vi "Get V.vi"(8 "error in (no error)":errorcluster, 10 "chan (0)":i32, 11 "VISA resource name":refnum<visa-resource-name>) -> (0 "error out":errorcluster, 2 "output":string, 3 "VISA resource name out":refnum<visa-resource-name>)   [LabVIEW 2023]
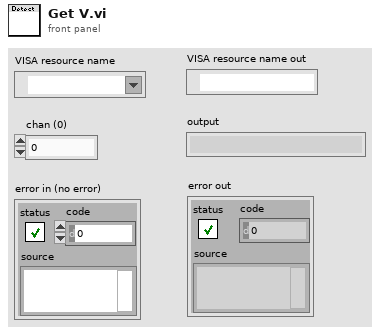
[diagram p1: front panel]
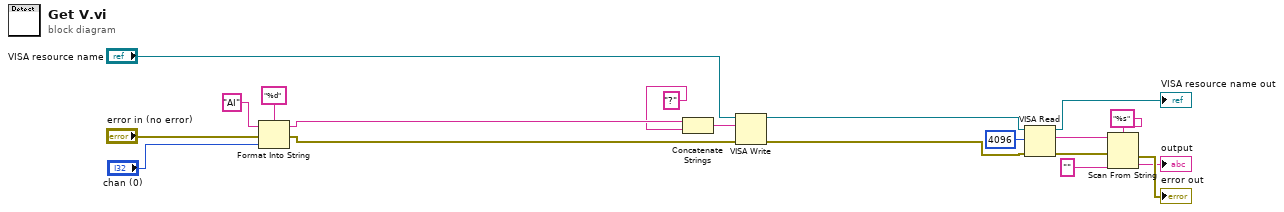
[diagram p0: block diagram]
diagram:
  n1 = Format Into String(format string="%d", initial string="AI" ("command"), error in="error in (no error)", "chan (0)") -> (resulting string=w11:string, error out=w17:errorcluster)
  n2 = Concatenate Strings(w11, "?" ("command")) -> (w12:string)
  n3 = VISA Write(VISA resource name="VISA resource name", write buffer=w12, error in (no error)=w17) -> (VISA resource name out=w1:refnum<visa-resource-name>, error out=w13:errorcluster)  [unwired: 1 out]
  n4 = VISA Read(VISA resource name=w1, byte count=u32 4096, error in (no error)=w13) -> (VISA resource name out=→"VISA resource name out":refnum<visa-resource-name>, read buffer=w7:string, error out=w5:errorcluster)  [unwired: 1 out]
  n5 = Scan From String(format string="%s", input string=w7, error in=w5, default 1="" ("default value 1")) -> (error out=→"error out":errorcluster, output 1=→"output":string)  [unwired: 1 in, 2 out]
